vi "[subVI]_convert_ascii_string_to_hex.vi"(11 "input (ascii data)":string) -> (3 "output (hex data)":string)   [LabVIEW 2013]
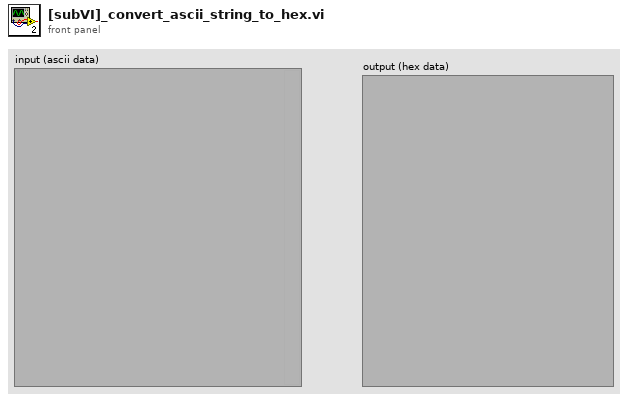
[diagram p1: front panel]
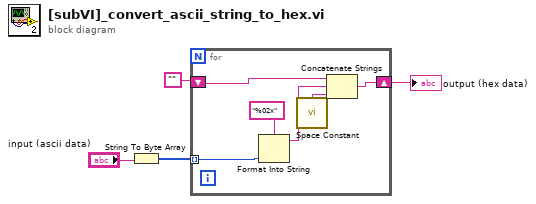
[diagram p0: block diagram]
diagram:
  n1 = String To Byte Array(string="input (ascii data)") -> (unsigned byte array=w4:u8[])
  n2 = for {
    tunnel: w4 -> [w10] mode=indexing
    shift-right: [w8] -> w2
    shift-left: "" -> [w7]
    n3 = Format Into String(format string="%02x", w10) -> (resulting string=w6:string)  [unwired: 2 in, 1 out]
    n4 = call <vilib>:"Space Constant.vi"() -> ("String"=w5:string)
    n5 = Concatenate Strings(w7, w6, w5) -> (w8:string)
  }
  "output (hex data)" <- w2
